vi "Get New Goal.vi"(11 "Obstacle Avoidance Data":T1={"dt"=100.0, "Wall Left?"=TRUE, "Encoder-Estimated Absolute Position"={"X"=-0.02048928758671903, "Y"=0.0}, "Wall Distance"=0.0, "Lidar Points"=[{"X"=-323.1806499880408, "Y"=-88.12504508331583}, {"X"=-272.24993117699097, "Y"=-193.4549511903018}, {"X"=-189.54344323151335, "Y"=-276.2073776854885}, {"X"=-83.32736349180192, "Y"=-326.5304510104155}, {"X"=34.520665924667675, "Y"=-338.24508542181394}, {"X"=148.01460731851458, "Y"=-303.87783898838}, {"X"=243.60760386956852, "Y"=-234.3273727280372}, {"X"=309.40297285322765, "Y"=-136.11200851782294}, {"X"=337.352070547106, "Y"=-21.246276966855408}, {"X"=324.0359279086246, "Y"=96.21847813812283}, {"X"=268.67760306496837, "Y"=200.12085152928722}, {"X"=184.9723383230988, "Y"=282.9077827461541}, {"X"=76.23632097390332, "Y"=329.2949240428146}, {"X"=-41.946856345804896, "Y"=336.3922441146458}, {"X"=-155.22172508685856, "Y"=301.36498614822324}, {"X"=-249.50605857482313, "Y"=229.47222470675726}, {"X"=-313.266202989234, "Y"=129.50848791584534}, {"X"=-339.7016632210197, "Y"=13.742601461119166}, {"X"=-322.70331116300844, "Y"=-103.78029014569411}, {"X"=-267.22584836266697, "Y"=-208.56748311404297}, {"X"=-178.52831165939736, "Y"=-286.99185647051775}, {"X"=-68.3704301970119, "Y"=-328.9660805190273}, {"X"=49.09710280636483, "Y"=-332.3965794130988}, {"X"=160.56117107635004, "Y"=-295.1655289677286}, {"X"=252.38655093062602, "Y"=-221.82734486708733}, {"X"=314.2728881686838, "Y"=-121.71454225964898}, {"X"=337.9659743006086, "Y"=-6.070350839399263}, {"X"=319.38622252224684, "Y"=110.67758777407415}, {"X"=261.73896426660167, "Y"=213.88651162394208}, {"X"=172.07609772102572, "Y"=290.9310358256732}, {"X"=61.18444452726066, "Y"=331.40303344936234}, {"X"=-56.1755041559914, "Y"=329.2385310392593}, {"X"=-166.11659933914768, "Y"=289.74897373870476}, {"X"=-255.73440648415715, "Y"=214.81488144163671}, {"X"=-316.8872577929115, "Y"=114.6232081228011}, {"X"=-335.97609469823783, "Y"=-1.5151072096523177}, {"X"=-314.90337845373676, "Y"=-117.12795365259899}, {"X"=-255.3065221325193, "Y"=-218.4127222468441}, {"X"=-164.4759151786029, "Y"=-292.9794069857057}, {"X"=-53.52272249238834, "Y"=-331.7063829236404}, {"X"=64.17068350767795, "Y"=-330.83795517069166}, {"X"=174.17605221655685, "Y"=-288.5114207460314}, {"X"=265.99720707069446, "Y"=-213.39490527499729}, {"X"=329.8492068633112, "Y"=-110.9820573892598}, {"X"=347.893847182183, "Y"=9.38759112542466}, {"X"=319.6668698793097, "Y"=127.13060754441236}, {"X"=256.3365992941863, "Y"=229.429840585493}, {"X"=161.18172537501965, "Y"=302.78054095792004}, {"X"=47.057356582408424, "Y"=339.7595224788988}, {"X"=-72.82095800488626, "Y"=335.1762574472391}, {"X"=-183.2528063931194, "Y"=288.74711962257294}, {"X"=-270.68363356252587, "Y"=207.36508354096443}, {"X"=-326.49024889938465, "Y"=101.75823233821939}, {"X"=-340.56268918928714, "Y"=-16.85522288757691}, {"X"=-314.84750279158754, "Y"=-133.4996163441268}, {"X"=-251.80602966629917, "Y"=-235.81434297253455}, {"X"=-156.09682732370482, "Y"=-309.8973756811919}, {"X"=-40.17470622072572, "Y"=-347.6842623099995}, {"X"=82.01414719192236, "Y"=-340.26025342885225}, {"X"=194.17284574471853, "Y"=-291.2127443676578}, {"X"=278.5446112506199, "Y"=-203.59104470659167}, {"X"=331.61856526734056, "Y"=-95.22455569087927}, {"X"=344.1286496103069, "Y"=24.790603044562847}, {"X"=318.19118088246313, "Y"=143.41691326352705}, {"X"=249.34273340661073, "Y"=244.2118313830306}, {"X"=151.284268952251, "Y"=317.8415784027632}, {"X"=32.578773735604415, "Y"=350.4910242984861}, {"X"=-89.5974227158357, "Y"=338.33212949429856}, {"X"=-200.62581107509126, "Y"=286.7770251445712}, {"X"=-287.10945394876205, "Y"=200.1409395828128}, {"X"=-338.4689436968192, "Y"=89.02192852266987}, {"X"=-353.39929842597405, "Y"=-33.45823743865886}, {"X"=-321.16300539925976, "Y"=-153.5485680191921}, {"X"=-247.94280515245723, "Y"=-254.045674260437}, {"X"=-145.70117751034908, "Y"=-324.8094761943244}, {"X"=-24.93516003204951, "Y"=-355.1242255423239}, {"X"=98.883642670153, "Y"=-341.9971884434946}, {"X"=210.01713189707039, "Y"=-286.2278988721134}, {"X"=301.5708528836656, "Y"=-200.27825197727435}, {"X"=349.1778649387704, "Y"=-83.48728662723555}, {"X"=356.5720420463536, "Y"=41.856782309588134}, {"X"=320.3498300197477, "Y"=162.08057707849864}, {"X"=246.9889347547002, "Y"=264.6707141781224}, {"X"=141.51738767491017, "Y"=335.37237177019733}, {"X"=17.6106304153272, "Y"=368.58050265187137}, {"X"=-110.6907593722161, "Y"=353.04818285920595}, {"X"=-225.49668647224283, "Y"=293.329172496208}, {"X"=-317.7868467837357, "Y"=200.93406167011483}, {"X"=-367.54310160260786, "Y"=79.20231468780214}, {"X"=-374.3165010260449, "Y"=-52.495882533129254}, {"X"=-335.1065478161003, "Y"=-179.13645358246876}, {"X"=-260.9080211496034, "Y"=-292.54112948614454}, {"X"=-144.20756224329773, "Y"=-364.5027697447641}, {"X"=-9.863913254201814, "Y"=-391.8753610351024}, {"X"=125.68887910921369, "Y"=-371.31045743372164}, {"X"=245.86885553642853, "Y"=-305.32373116542277}, {"X"=330.83243445790504, "Y"=-198.89559304476884}, {"X"=378.10924632585085, "Y"=-72.62156567618513}, {"X"=379.99208259095053, "Y"=62.020869733526695}, {"X"=335.39359309761153, "Y"=189.0763899613866}, {"X"=257.55382363169826, "Y"=302.13503885118}, {"X"=138.10416378391602, "Y"=373.27858073775377}, {"X"=1.1252397726958596, "Y"=401.99848199510114}, {"X"=-136.009467007011, "Y"=374.0318849917609}, {"X"=-262.9379100296832, "Y"=311.9565358002605}, {"X"=-354.28122867574706, "Y"=202.32224951356753}, {"X"=-404.25545470552566, "Y"=68.27123192441968}, {"X"=-403.0384689599272, "Y"=-75.12307352890211}, {"X"=-356.815140974168, "Y"=-211.88046860363576}, {"X"=-260.7624485821067, "Y"=-320.25186855981286}, {"X"=-134.52828046366326, "Y"=-390.46847319396363}, {"X"=8.204467320581063, "Y"=-414.91929637407253}, {"X"=150.58764987119767, "Y"=-386.722807904821}, {"X"=276.5367556308213, "Y"=-313.46890507289135}, {"X"=372.8474789421793, "Y"=-201.93076978284986}, {"X"=419.5817315820402, "Y"=-61.191208227447824}, {"X"=415.9704248697036, "Y"=87.23904566897099}, {"X"=362.1834006997155, "Y"=226.20129442045766}, {"X"=262.7500012795225, "Y"=337.8715784561928}, {"X"=130.9380773190073, "Y"=409.58587029344073}, {"X"=-18.285212865076094, "Y"=433.61376969452664}, {"X"=-166.87069128919308, "Y"=401.711754677018}, {"X"=-294.9984557589688, "Y"=319.6698641780571}, {"X"=-393.26552956414827, "Y"=201.71789056936117}, {"X"=-439.667637620544, "Y"=54.06802249037355}, {"X"=-431.3936031681613, "Y"=-100.65227682761729}, {"X"=-378.7057661555241, "Y"=-248.5466222623828}, {"X"=-269.95047650255594, "Y"=-363.76459095180996}, {"X"=-128.1700643736734, "Y"=-434.48381092052165}, {"X"=29.29169601622637, "Y"=-452.05331152049894}, {"X"=185.59861368568238, "Y"=-419.8115764779301}, {"X"=318.81635396902715, "Y"=-330.227492286776}, {"X"=413.936115475137, "Y"=-200.68346817256304}, {"X"=465.6878120203884, "Y"=-46.668453358395816}, {"X"=461.0245949085407, "Y"=118.5378192840763}, {"X"=392.83084923010824, "Y"=270.6086124309917}, {"X"=276.19450560659703, "Y"=390.1434514511643}, {"X"=125.21208864864042, "Y"=462.35058499954494}, {"X"=-41.92365225064198, "Y"=480.171520386852}, {"X"=-208.9600861346141, "Y"=445.411179806037}, {"X"=-349.56204540353554, "Y"=346.202327315878}, {"X"=-448.3095160191909, "Y"=205.05903135835}, {"X"=-491.50295053647517, "Y"=38.127524224919625}, {"X"=-474.5690978380277, "Y"=-133.4680628163115}, {"X"=-399.5794494181969, "Y"=-288.7367122247082}, {"X"=-282.97808506336145, "Y"=-419.4613294635524}, {"X"=-122.65847750604645, "Y"=-497.08537607381555}, {"X"=56.78964147629118, "Y"=-515.8859014935141}, {"X"=231.86051199402908, "Y"=-466.5738996895093}, {"X"=379.0781586926409, "Y"=-358.8861703454295}, {"X"=483.1553171646294, "Y"=-207.98254275832946}, {"X"=527.2236794009434, "Y"=-28.99648830979267}, {"X"=509.7447457217066, "Y"=155.78890333616079}, {"X"=424.9195931833705, "Y"=321.7914720879966}, {"X"=288.1172033706664, "Y"=448.42979755423505}, {"X"=116.07239687935517, "Y"=520.2124131009483}, {"X"=-71.09066773783442, "Y"=535.2973036981467}, {"X"=-256.65893808742067, "Y"=488.69179608669333}, {"X"=-415.92062302877827, "Y"=376.4491879191998}, {"X"=-521.0430563482452, "Y"=210.56301054414882}, {"X"=-572.6773798182919, "Y"=18.605126217947753}, {"X"=-545.0052456719017, "Y"=-180.0637338051987}, {"X"=-449.66150020298033, "Y"=-356.7381509283883}, {"X"=-304.00218356953457, "Y"=-497.4527257828746}, {"X"=-114.29723947149002, "Y"=-572.7018918175198}, {"X"=92.37631379621854, "Y"=-592.8493920713175}, {"X"=291.8536627008311, "Y"=-526.5333787097977}, {"X"=462.8868427108885, "Y"=-400.37324944183655}, {"X"=573.3859278495552, "Y"=-216.84343167972972}, {"X"=625.9891548532436, "Y"=-6.263364108117484}, {"X"=596.4547994819278, "Y"=212.02620975483342}, {"X"=487.72918257570166, "Y"=405.08792933287884}, {"X"=322.9202889249307, "Y"=556.0438106787658}, {"X"=111.86192933358328, "Y"=634.2140744957003}, {"X"=-114.96478358236187, "Y"=642.7965362562429}, {"X"=-336.34875491818013, "Y"=575.9728566108312}, {"X"=-517.974105643847, "Y"=428.09531604751277}, {"X"=-638.4277610328531, "Y"=225.19509688882846}, {"X"=-688.925990260344, "Y"=-8.587684118125615}, {"X"=-644.7642936053695, "Y"=-245.66762861574412}, {"X"=-526.0101162810365, "Y"=-457.2754115465946}, {"X"=-341.67497755214754, "Y"=-620.087258328355}, {"X"=-108.29947213398765, "Y"=-706.7473282281502}, {"X"=145.27187083916175, "Y"=-718.4643596987667}, {"X"=384.84892969249677, "Y"=-626.2044965149361}, {"X"=587.9434258312447, "Y"=-464.0556224052049}, {"X"=725.092239633645, "Y"=-237.570951191646}, {"X"=767.5519052771331, "Y"=26.823971910998935}, {"X"=719.7053279452265, "Y"=292.8868945622645}, {"X"=585.1831925331331, "Y"=532.2270293120829}, {"X"=371.2027607596003, "Y"=710.9344001698585}, {"X"=104.58339973567159, "Y"=802.2141844661099}, {"X"=-180.92844554321317, "Y"=801.836319321842}, {"X"=-456.2944746576037, "Y"=706.4401274557524}, {"X"=-673.2550281135017, "Y"=507.29584826637074}, {"X"=-825.9106062278732, "Y"=250.21355970576826}, {"X"=-872.5398953854548, "Y"=-50.143544940837444}, {"X"=-815.6657221729646, "Y"=-353.52086845493665}, {"X"=-661.4219637873729, "Y"=-629.335269367751}, {"X"=-410.88602605945636, "Y"=-832.06960985566}, {"X"=-101.14234449664634, "Y"=-940.5753989238416}, {"X"=236.20640958236856, "Y"=-946.9911356789497}, {"X"=-172.8577138849469, "Y"=463.8298468919785}, {"X"=-321.36002564402054, "Y"=375.16738214068533}, {"X"=-429.1530070449495, "Y"=240.57038480599917}, {"X"=-487.72167179357893, "Y"=78.38102004869708}, {"X"=-482.9178355608517, "Y"=-93.9924166759435}, {"X"=-421.01158030760183, "Y"=-254.5505772383797}, {"X"=-309.4768776048346, "Y"=-386.3112474244802}, {"X"=-157.51458139905935, "Y"=-469.26293429563924}, {"X"=13.718731556429965, "Y"=-494.8104264854815}, {"X"=183.27636013856727, "Y"=-459.82853956518267}, {"X"=326.41178586595856, "Y"=-364.12871559091474}, {"X"=431.8415623152359, "Y"=-229.45927937054472}, {"X"=486.42864386816825, "Y"=-66.99333666502285}, {"X"=479.7480436239394, "Y"=104.6062790202471}, {"X"=414.38312823248737, "Y"=263.40957356675153}, {"X"=298.32988470712866, "Y"=389.9903904001064}, {"X"=145.78492330161677, "Y"=468.86429782674804}, {"X"=-24.490920269000597, "Y"=488.38528929683093}, {"X"=-190.39259270695973, "Y"=448.2319245717981}, {"X"=-331.04949759187207, "Y"=353.05617653234026}, {"X"=-432.38010897426665, "Y"=217.4528055068301}, {"X"=-480.8158371070427, "Y"=55.248775726864764}, {"X"=-474.31964968131734, "Y"=-114.65353271033915}, {"X"=-407.4876256248847, "Y"=-272.0976594542555}, {"X"=-289.45131519617297, "Y"=-396.594344902844}, {"X"=-134.8973836368717, "Y"=-471.05962209208684}, {"X"=35.571282929362404, "Y"=-488.70864640544255}, {"X"=202.1026496042253, "Y"=-447.4860897075577}, {"X"=344.54131725503396, "Y"=-351.2398028365018}, {"X"=445.3269813384388, "Y"=-211.54462445868114}, {"X"=490.93875895350584, "Y"=-45.257623757991624}, {"X"=476.4972788638774, "Y"=126.56567068155258}, {"X"=403.76914455336737, "Y"=282.9063862323964}, {"X"=281.65107399318293, "Y"=404.6396097249798}, {"X"=124.57423094691966, "Y"=474.93932816588284}, {"X"=-46.59655729874159, "Y"=488.78200761440485}, {"X"=-212.0647557548933, "Y"=442.8327549259102}, {"X"=-351.5889006630543, "Y"=342.71246971555917}, {"X"=-448.1012234190961, "Y"=200.6687085741801}, {"X"=-489.79552378913553, "Y"=34.07746078604305}, {"X"=-471.5714037646752, "Y"=-136.68242903674175}, {"X"=-399.6875056725075, "Y"=-293.6826838017205}, {"X"=-970.6876197700103, "Y"=23.806868963058022}, {"X"=-908.1493198505384, "Y"=-308.07239047019635}, {"X"=-732.5003439418726, "Y"=-590.6726918394132}, {"X"=-478.62775897293136, "Y"=-797.3680796452397}, {"X"=-171.0069858495901, "Y"=-893.7838680286204}, {"X"=145.94754460362194, "Y"=-890.1175734288088}, {"X"=435.6800686635159, "Y"=-771.4899421884827}, {"X"=664.0465806219879, "Y"=-565.2020435447465}, {"X"=799.3052855670975, "Y"=-295.0386660023074}, {"X"=838.018727584477, "Y"=-1.718316416824205}, {"X"=784.5363346403902, "Y"=285.93686084584493}, {"X"=613.6325642279008, "Y"=517.9664289193291}, {"X"=395.75074662043465, "Y"=694.1171107466505}, {"X"=130.85819628289016, "Y"=778.076149504797}, {"X"=-143.06366443365985, "Y"=764.7293148257588}, {"X"=-396.12470118495685, "Y"=666.1035865880564}, {"X"=-582.6568140142175, "Y"=473.8018153373172}, {"X"=-704.5046255238351, "Y"=242.2175934979805}, {"X"=-729.8273293323049, "Y"=-14.90508825152121}, {"X"=-678.1907522557332, "Y"=-264.60066485983833}, {"X"=-537.3451435145912, "Y"=-474.6863982495337}, {"X"=-334.82884436472125, "Y"=-619.267247440558}, {"X"=-100.08858571130943, "Y"=-689.7732765937409}, {"X"=142.33268393343045, "Y"=-676.1865417583253}, {"X"=359.0586381589263, "Y"=-573.9517468002357}, {"X"=534.7473369562654, "Y"=-415.2062118782881}, {"X"=644.0710063407504, "Y"=-205.36536096321763}, {"X"=669.4043569377037, "Y"=28.726951278732585}, {"X"=616.7230445567536, "Y"=256.71376730608006}, {"X"=490.59964198567553, "Y"=453.3829451336091}, {"X"=297.1723940707359, "Y"=580.3488136317212}, {"X"=78.78134937438514, "Y"=644.2031720803521}, {"X"=-147.4213529932607, "Y"=629.9761131541653}, {"X"=-353.14800815946495, "Y"=537.3276583342717}, {"X"=-511.76309205597244, "Y"=379.2710981173764}, {"X"=-610.1086819551149, "Y"=179.5505343871025}, {"X"=-626.6386416154863, "Y"=-41.01626087059915}, {"X"=-560.4698605784341, "Y"=-248.2328900590442}, {"X"=-439.9861867024582, "Y"=-425.36822293654194}, {"X"=-266.15588941510975, "Y"=-549.9737588473824}, {"X"=-59.79044755359907, "Y"=-601.0313235050064}, {"X"=149.84326946937585, "Y"=-580.9932310609129}, {"X"=336.778086995805, "Y"=-488.10175208227827}, {"X"=473.64997776549814, "Y"=-334.7762053135676}, {"X"=553.2081006293536, "Y"=-149.3735808568249}, {"X"=570.8118733902091, "Y"=50.261275692252106}, {"X"=517.6866255968064, "Y"=243.32236090972924}, {"X"=402.2322412780878, "Y"=406.7059214724217}, {"X"=237.16062095307385, "Y"=519.4281066265817}, {"X"=43.09340984535263, "Y"=560.3469670789915}, {"X"=-150.3339007821096, "Y"=533.2068617213863}, {"X"=-323.5829819907349, "Y"=447.1965936549836}, {"X"=-455.30086172822706, "Y"=306.73028430387194}, {"X"=-529.1945660028812, "Y"=130.2168393638356}, {"X"=-536.6980706417138, "Y"=-59.44062102146838}, {"X"=-483.40082429271774, "Y"=-240.63215407815508}, {"X"=-366.1583086417559, "Y"=-387.3010301393757}, {"X"=-205.65113244726987, "Y"=-478.6858928493236}, {"X"=-28.12020471154562, "Y"=-518.2365303037284}, {"X"=151.47769540755118, "Y"=-494.3174230333527}, {"X"=313.0439247297058, "Y"=-412.7230655827385}, {"X"=436.02553688412684, "Y"=-279.68481987826726}, {"X"=506.64749912825664, "Y"=-112.6502237010726}, {"X"=513.4616704786683, "Y"=68.57224990553341}, {"X"=461.0985116417334, "Y"=242.5861853073852}, {"X"=349.3588079184538, "Y"=386.5277986589823}, {"X"=185.90860989445582, "Y"=460.92798419844945}, {"X"=15.811371406642953, "Y"=496.74907955818304}, {"X"=-156.21754078711183, "Y"=471.8036434348272}, {"X"=-307.26797687522094, "Y"=386.7942587000343}, {"X"=-421.67138622063067, "Y"=257.3168516253105}, {"X"=-475.6627812455304, "Y"=94.60669180833496}, {"X"=-478.15926279347514, "Y"=-74.83398091571925}, {"X"=-422.2672578975743, "Y"=-234.43988265071604}, {"X"=-314.3980798519114, "Y"=-364.0081913642475}, {"X"=-168.75591150484374, "Y"=-447.2119481135906}, {"X"=-4.419315035715807, "Y"=-476.9793372228726}, {"X"=159.43608343540618, "Y"=-447.4501853195478}, {"X"=303.77180815581437, "Y"=-365.185071280046}, {"X"=394.5129281311917, "Y"=-228.71754566544428}, {"X"=445.2067614451207, "Y"=-78.18684724733478}, {"X"=440.9651145927378, "Y"=79.1949330102621}, {"X"=386.72310866076896, "Y"=226.1970030082622}, {"X"=285.1763811666914, "Y"=345.5287503618655}, {"X"=147.75104679353345, "Y"=419.7626500523625}, {"X"=-5.770599802310607, "Y"=439.9618884484801}, {"X"=-156.2105539392829, "Y"=409.18927299263845}, {"X"=-286.90874544352175, "Y"=329.6067569947868}, {"X"=-379.35936428225335, "Y"=208.71014998156343}, {"X"=-430.9930882559745, "Y"=65.75177543687005}, {"X"=-426.29307203090286, "Y"=-86.49709495668866}, {"X"=-368.7281265738194, "Y"=-226.96576459963546}, {"X"=-267.3957876803396, "Y"=-339.2823821135034}, {"X"=-134.2024507971371, "Y"=-410.61929126018015}, {"X"=15.410166664633435, "Y"=-431.7257900916164}, {"X"=160.87463777664524, "Y"=-394.4641211997105}, {"X"=286.8758201049923, "Y"=-314.9444699969136}, {"X"=377.78644221184584, "Y"=-196.89815847596552}, {"X"=416.53533893156646, "Y"=-53.99425919533432}, {"X"=409.6532782010828, "Y"=92.74145915905774}, {"X"=353.50110584863256, "Y"=228.6754331265667}, {"X"=253.13289097983008, "Y"=336.4150890040226}, {"X"=120.35550091927436, "Y"=398.2153751120135}, {"X"=-24.136195803950898, "Y"=415.29803101554467}, {"X"=-164.0796382158633, "Y"=377.9089151546328}, {"X"=-281.4220064948224, "Y"=295.3880863673561}, {"X"=-367.7230340927278, "Y"=181.28624054746152}, {"X"=-405.67027614102926, "Y"=43.34746643050395}, {"X"=-393.8436600277698, "Y"=-98.52427053315635}, {"X"=-334.9977384111693, "Y"=-227.56930177329377}, {"X"=-234.3903395534906, "Y"=-326.5816334732239}, {"X"=-107.05407735948715, "Y"=-385.4024353547099}, {"X"=32.214224676893444, "Y"=-398.7023493806919}, {"X"=167.54431783559977, "Y"=-363.2296337974311}, {"X"=282.3814852486064, "Y"=-283.3236099584731}, {"X"=362.6778773351193, "Y"=-168.75905574084422}, {"X"=399.60743927053164, "Y"=-33.634348564041886}, {"X"=386.7495163300058, "Y"=106.02669306747188}, {"X"=326.5836414188409, "Y"=232.71765654994755}, {"X"=225.90509960198176, "Y"=330.1153477545597}, {"X"=98.4088215967465, "Y"=387.71089237397285}, {"X"=-40.81456866821461, "Y"=394.89428717284113}, {"X"=-173.86565178493896, "Y"=355.7802832408026}, {"X"=-283.58346093628154, "Y"=272.0621241875055}, {"X"=-359.0098715991871, "Y"=157.35691901379164}, {"X"=-391.23830298910207, "Y"=24.094760139642897}, {"X"=-375.60466337112865, "Y"=-112.11487274272211}, {"X"=-312.4191367316311, "Y"=-233.41268194545756}, {"X"=-210.1996861000159, "Y"=-322.5406607855909}, {"X"=-84.92518281517638, "Y"=-369.35786547873846}, {"X"=47.33925008646465, "Y"=-375.0265788933613}, {"X"=173.59112254468602, "Y"=-335.79344137539306}, {"X"=277.13635262385475, "Y"=-254.13145867325207}, {"X"=349.5501626686048, "Y"=-143.92014253105364}, {"X"=377.73253845963126, "Y"=-14.751539250364072}, {"X"=359.709994962293, "Y"=116.22159656228018}, {"X"=302.41206994720744, "Y"=236.67558375585787}, {"X"=202.4137025366019, "Y"=326.3326328008565}, {"X"=76.24164560774277, "Y"=369.21448418123896}, {"X"=-55.564965549426205, "Y"=372.8796819492347}, {"X"=-180.57189567978907, "Y"=330.93109629014185}, {"X"=-281.2312144587987, "Y"=246.52277610751395}, {"X"=-351.72153874050724, "Y"=135.6707253562225}, {"X"=-373.92819735851174, "Y"=6.195139680270765}, {"X"=-353.1893110713746, "Y"=-122.95867976837864}, {"X"=-289.24282695086373, "Y"=-237.07115783817778}, {"X"=-190.41905633825434, "Y"=-323.0445471785946}, {"X"=-67.34556199141798, "Y"=-367.88288236213776}, {"X"=63.46087637754713, "Y"=-368.58013685747636}, {"X"=185.01087313052508, "Y"=-321.58911344391356}, {"X"=280.60701877535416, "Y"=-235.00467967683156}, {"X"=342.49088317566265, "Y"=-123.32894757576635}, {"X"=364.01414412311993, "Y"=2.1492416036112623}, {"X"=341.01063532622084, "Y"=127.36451744717198}, {"X"=273.2583633588584, "Y"=234.39510270697184}, {"X"=177.78189973253225, "Y"=317.6426938505333}, {"X"=56.89227797095047, "Y"=355.47939413129814}, {"X"=-69.00095791539245, "Y"=353.32143980518134}, {"X"=-183.86102848657336, "Y"=303.6652555381851}, {"X"=-277.18579419776205, "Y"=221.76942168892552}, {"X"=-336.6003524301472, "Y"=112.74488423535826}, {"X"=-354.83661397741724, "Y"=-10.071557097605567}, {"X"=-329.66376572476645, "Y"=-131.6559607345968}, {"X"=-264.1611624990307, "Y"=-237.1350983285571}, {"X"=-166.34163444914785, "Y"=-313.6058733279774}, {"X"=-47.899787188147705, "Y"=-349.73225058963203}, {"X"=75.4668205180852, "Y"=-344.8432268493292}, {"X"=189.60419751073667, "Y"=-297.7700750182253}, {"X"=280.5500984675005, "Y"=-214.27117952110322}, {"X"=337.1792547544368, "Y"=-104.56082855864138}, {"X"=352.5643109923841, "Y"=17.940283659297304}, {"X"=324.82323751541156, "Y"=138.24678927068152}, {"X"=257.3495560917175, "Y"=241.64178317856204}, {"X"=158.3972157576234, "Y"=315.4771188416605}, {"X"=39.957442994353336, "Y"=349.7270932150147}, {"X"=-82.44784741152864, "Y"=340.14551803909063}, {"X"=-194.53800173950813, "Y"=290.9415638393041}, {"X"=-282.82812269688617, "Y"=206.14718697682272}, {"X"=-334.5947429811157, "Y"=95.58580613125747}, {"X"=-347.0446874038669, "Y"=-25.490451705101734}, {"X"=-317.03869611585037, "Y"=-143.44850278517686}, {"X"=-253.24124812283122, "Y"=-248.7639289846028}, {"X"=-150.79966487582675, "Y"=-318.05232446584034}, {"X"=-32.322047272168916, "Y"=-353.52363475287035}, {"X"=90.62518177910192, "Y"=-340.13936805156493}, {"X"=202.2155644795054, "Y"=-288.1339125617364}, {"X"=289.0717425120243, "Y"=-200.88148996207207}, {"X"=339.6012699864925, "Y"=-88.8025527781811}, {"X"=349.41158444140046, "Y"=33.56877458619342}, {"X"=316.48143724822893, "Y"=151.83368669650255}, {"X"=243.44414341859328, "Y"=250.0918323526542}, {"X"=142.43241416541437, "Y"=318.6217877870124}, {"X"=23.999658738713897, "Y"=348.1752424174271}, {"X"=-97.36643066957394, "Y"=335.13696874749223}, {"X"=-206.22666750403232, "Y"=280.29646861024366}, {"X"=-290.96984372409077, "Y"=192.6801133842127}, {"X"=-339.52396718185736, "Y"=80.68805413981538}, {"X"=-346.5421527727432, "Y"=-41.17444751497799}, {"X"=-309.3825739635234, "Y"=-157.09469899022545}, {"X"=-236.36023871677946, "Y"=-254.03376041015858}, {"X"=-134.03437998882404, "Y"=-318.97537839664744}, {"X"=-15.991012991853408, "Y"=-345.62932716243205}, {"X"=104.01101582734047, "Y"=-330.0029854258667}, {"X"=211.29204753760897, "Y"=-274.00789892739857}, {"X"=292.7285627219488, "Y"=-184.49385828895257}, {"X"=338.3585609107794, "Y"=-72.41097492990498}, {"X"=347.55077019042534, "Y"=49.23112689746266}, {"X"=310.2221244483157, "Y"=166.36990576306158}, {"X"=233.956887133269, "Y"=263.01665681661046}, {"X"=129.80784108365987, "Y"=329.3497279697713}, {"X"=8.476749347705148, "Y"=354.89926974536826}, {"X"=-114.89922218981273, "Y"=337.997721758522}, {"X"=-223.00838685241817, "Y"=276.1939905351424}, {"X"=-304.47858874142804, "Y"=182.49742869279007}, {"X"=-347.717587686466, "Y"=66.28898718782608}, {"X"=-348.2893664996788, "Y"=-57.351934243356666}, {"X"=-303.7536093627492, "Y"=-171.8205371577449}, {"X"=-226.00449970772678, "Y"=-265.9204850132242}, {"X"=-120.60610961122963, "Y"=-327.4907993182466}, {"X"=-0.4516579107484126, "Y"=-348.99968062596145}, {"X"=119.7605508118853, "Y"=-327.8159814074921}, {"X"=225.32514664940828, "Y"=-266.53107017957996}, {"X"=304.1976566993283, "Y"=-173.1365092213925}, {"X"=344.22881122773873, "Y"=-57.63359356438464}, {"X"=343.02258220276036, "Y"=64.4248729592119}, {"X"=301.5757114717766, "Y"=179.62585552599023}, {"X"=221.27443795186088, "Y"=272.48429349316035}, {"X"=113.90751782979441, "Y"=332.01015757025624}, {"X"=-7.454369141330379, "Y"=353.92107381656103}, {"X"=-128.8752618757328, "Y"=329.69968961472136}, {"X"=-234.5285406508528, "Y"=265.1466623492308}, {"X"=-311.48980649912676, "Y"=168.15866203937964}, {"X"=-350.34450914437286, "Y"=50.60007780402106}, {"X"=-346.3396140894595, "Y"=-73.14833414809861}, {"X"=-299.96503383036406, "Y"=-187.94862574557285}, {"X"=-215.0554418118153, "Y"=-277.3866324495924}, {"X"=-105.77194019158121, "Y"=-332.5792565162405}, {"X"=15.227478601480879, "Y"=-348.66853525376666}, {"X"=134.36665037460355, "Y"=-322.10574195624224}, {"X"=237.07146813827868, "Y"=-256.1402612357706}, {"X"=310.7782135104768, "Y"=-158.84154631521997}, {"X"=348.455843204178, "Y"=-42.35332502909006}, {"X"=342.70260775655606, "Y"=80.45474306477679}, {"X"=294.03691588203293, "Y"=193.54157406777648}, {"X"=209.99949962237193, "Y"=283.7566126433429}, {"X"=99.44040824559677, "Y"=338.7103182874456}, {"X"=-23.280565022900152, "Y"=352.23012487295824}, {"X"=-143.15115706551396, "Y"=322.662175782261}, {"X"=-245.50778740468704, "Y"=253.6234715962272}, {"X"=-316.02848203744674, "Y"=152.68938314233966}, {"X"=-349.278499498568, "Y"=34.514003432950865}, {"X"=-339.7993225383053, "Y"=-87.88341988461379}, {"X"=-288.75052392466836, "Y"=-199.53020304797872}, {"X"=-202.37682268338432, "Y"=-286.7687711500773}, {"X"=-92.80425724157985, "Y"=-344.72099795602236}, {"X"=31.936839935024896, "Y"=-359.5863548041691}, {"X"=155.51779350053565, "Y"=-330.22051478141935}, {"X"=259.7233633008266, "Y"=-256.4749836324456}, {"X"=332.15989009854076, "Y"=-151.3552722204959}, {"X"=363.9663278096192, "Y"=-27.720509059082243}, {"X"=350.2895673834843, "Y"=99.03319105153562}, {"X"=294.762054926987, "Y"=213.5963704851632}, {"X"=203.17927158054354, "Y"=302.0306427785813}, {"X"=86.74439479640083, "Y"=353.51798287116634}, {"X"=-40.74235497112793, "Y"=365.73541054694135}, {"X"=-165.0881393114198, "Y"=331.11801636600103}]}) -> (3 "New Goal":cluster{i32, i32})   [LabVIEW 2017]
panel:
  out "XY Graph":cluster{dbl[], dbl[]}[](graph)
  out "Lidar Point Retaintion Ratio":dbl(slide) scale=0.0..1.0
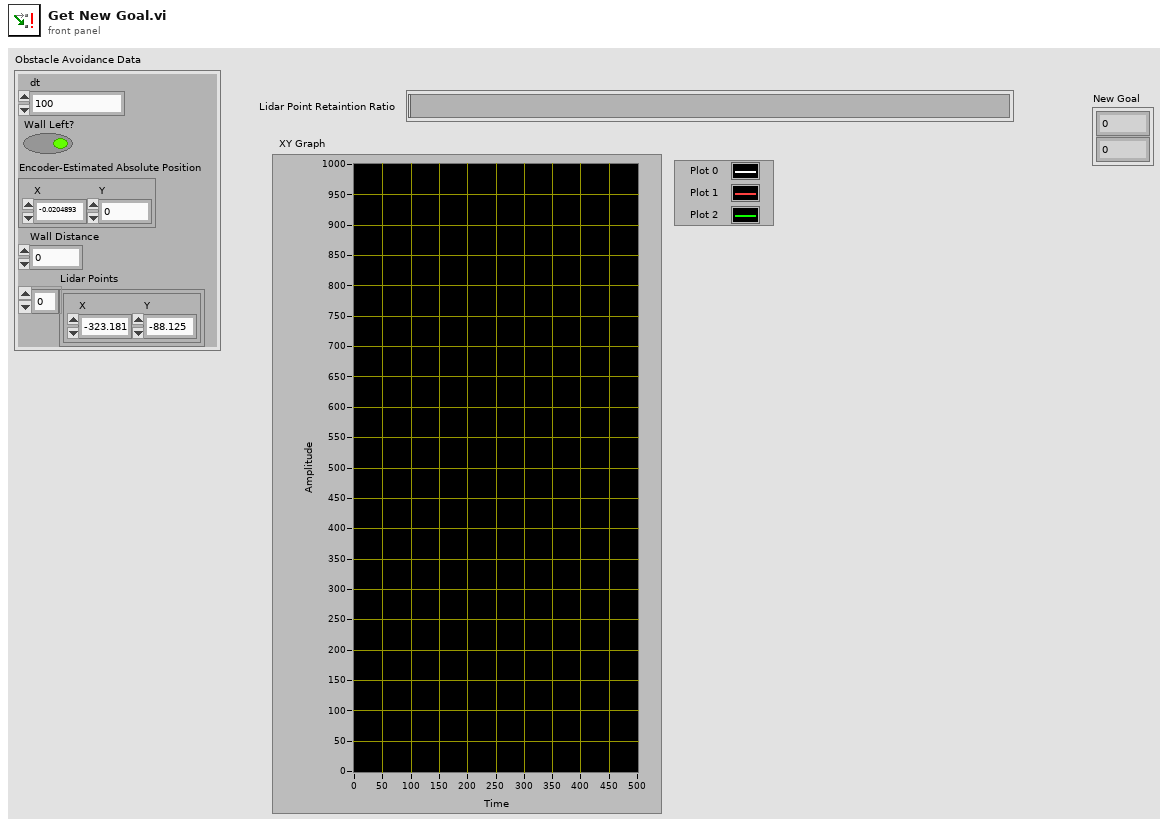
[diagram p1: front panel]
types:
  T1 = cluster{"dt":dbl, "Wall Left?":bool, "Encoder-Estimated Absolute Position":cluster{"X":dbl, "Y":dbl}, "Wall Distance":dbl, "Lidar Points":cluster{"X":dbl, "Y":dbl}[]}
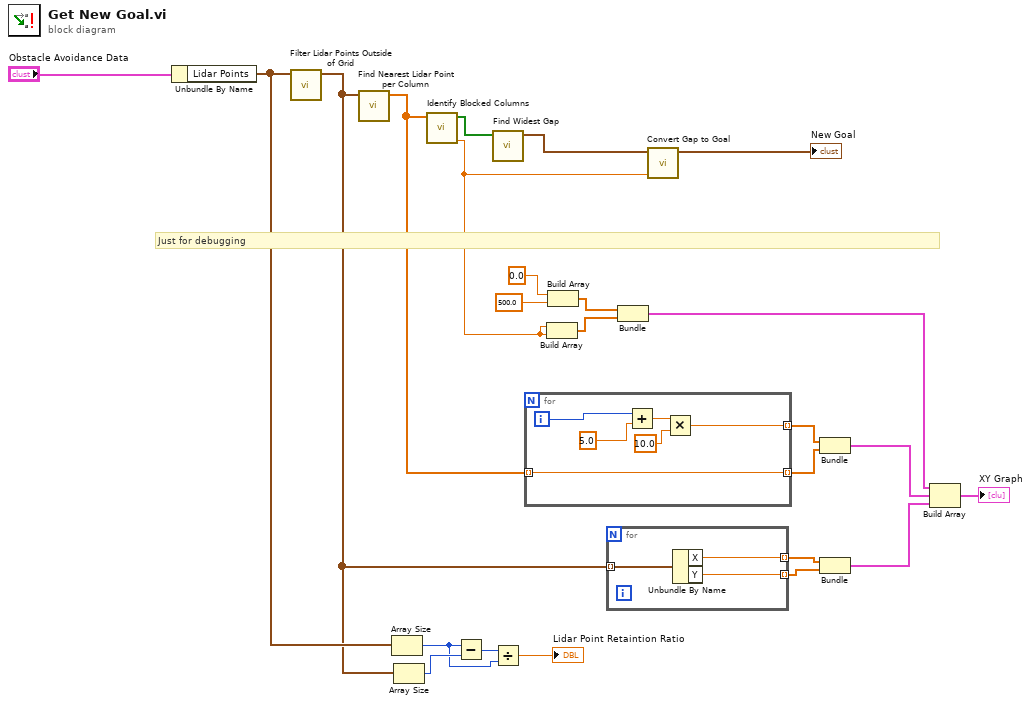
[diagram p0: block diagram]
diagram:
  # "Just for debugging"
  n1 = Unbundle By Name("Obstacle Avoidance Data") -> ("Lidar Points"=w20:cluster{"X":dbl, "Y":dbl}[])
  n2 = call "Filter Lidar Points Outside of Grid.vi"("Lidar Points"=w20) -> ("Filtered lidar points in the grid"=w15:cluster{"X":dbl, "Y":dbl}[])  [unwired: 10 in]
  n3 = call "Find Nearest Lidar Point per Column.vi"("Lidar Points"=w15) -> ("Nearest Point per Column"=w12:dbl[])  [unwired: 10 in]
  n4 = Array Size(array=w20) -> (size(s)=w17:i32)
  n5 = Array Size(array=w15) -> (size(s)=w18:i32)
  n6 = call "Identify Blocked Columns.vi"("Nearest Point per Column"=w12) -> ("Goal Y"=w4:dbl, "Blocked Columns"=w23:bool[])  [unwired: 9 in]
  n7 = Subtract(x=w17, y=w18) -> (x-y=w19:i32)
  n8 = call "Find Widest Gap.vi"("Blocked Columns"=w23) -> ("Best Known Gap (mm)"=w22:cluster{i32, i32})  [unwired: 10 in]
  n9 = Divide(x=w19, y=w17) -> (x/y=→"Lidar Point Retaintion Ratio":dbl)
  n10 = for {
    tunnel: w12 -> [w25] mode=indexing
    tunnel: [w26] -> w11 mode=indexing
    tunnel: [w25] -> w10 mode=indexing
    i -> [w30]
    n11 = Add(x=w30, y=5.0) -> (x+y=w28:dbl)
    n12 = Multiply(x=w28, y=10.0) -> (x*y=w26:dbl)
  }
  n13 = Build Array(w4, w4) -> (w3:dbl[])
  n14 = Build Array(0.0 ("element"), 500.0 ("element")) -> (w2:dbl[])
  n15 = for {
    tunnel: w15 -> [w33] mode=indexing
    tunnel: [w32] -> w14 mode=indexing
    tunnel: [w31] -> w13 mode=indexing
    n16 = Unbundle By Name(w33) -> ("X"=w32:dbl, "Y"=w31:dbl)
  }
  n17 = Bundle(w2, w3) -> (w1:cluster{dbl[], dbl[]})  [unwired: 1 in]
  n18 = call "Convert Gap to Goal.vi"("Goal Y"=w4, "Best Known Gap (mm)"=w22) -> ("Goal"=→"New Goal":cluster{"X":dbl, "Y":dbl})  [unwired: 9 in]
  n19 = Bundle(w11, w10) -> (w9:cluster{dbl[], dbl[]})  [unwired: 1 in]
  n20 = Bundle(w14, w13) -> (w8:cluster{dbl[], dbl[]})  [unwired: 1 in]
  n21 = Build Array(w1, w9, w8) -> (→"XY Graph":cluster{dbl[], dbl[]}[])
